vi "Make Up Setup Plot.vi"(4 "End Field":dbl format="%.2f", 5 "Start Field":dbl format="%.2f", 6 "Put in plot 1":bool, 7 "End X":i32, 8 "error in (no error)":errorcluster, 9 "Start X":i32, 10 "Plot 1 In":cluster{dbl[], dbl[]} {"?" format="%.2f"; "?" format="%.2f"}, 11 "Plot 2 In":cluster{dbl[], dbl[]} {"?" format="%.2f"; "?" format="%.2f"}) -> (0 "error out":errorcluster, 2 "Plot 1 Out":cluster{dbl[], dbl[]} {"?" format="%.2f"; "?" format="%.2f"}, 3 "Plot 2 Out":cluster{dbl[], dbl[]} {"?" format="%.2f"; "?" format="%.2f"})   [LabVIEW 2018, in "Multi Segment Waveform.xctl"]
doc: "Add a single ramp segment to one of two plots"
uses:
  Multi Segment Waveform.xctl
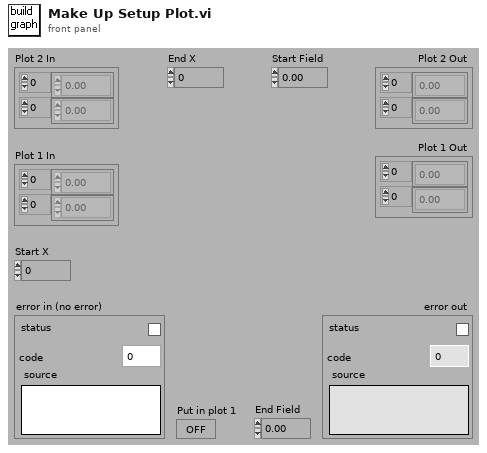
[diagram p1: front panel]
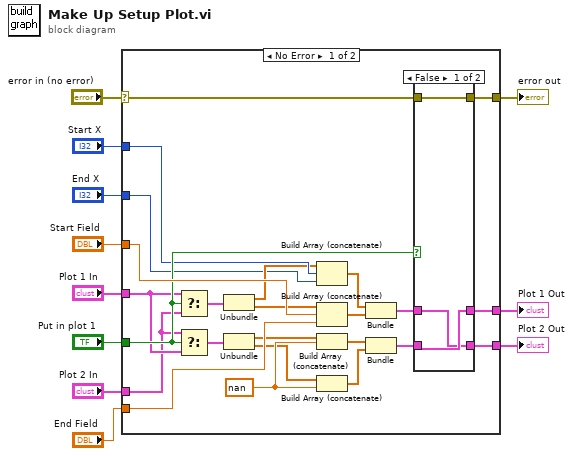
[diagram p0: block diagram]
diagram:
  n1 = case shown="No Error" "error in (no error)" {
    selector: "error in (no error)" -> [w13 w43]
    tunnel: [w35 w42] -> w11
    tunnel: [w34 _] -> w10
    tunnel: "End Field" -> [w33 _]
    tunnel: "Start Field" -> [w32 _]
    tunnel: "Put in plot 1" -> [w28 _]
    tunnel: "Plot 1 In" -> [w21 w42]
    tunnel: "Plot 2 In" -> [w20 _]
    tunnel: "Start X" -> [w17 _]
    tunnel: "End X" -> [w14 _]
    tunnel: [w12 w43] -> w1
    frame No Error {
      w25 = nan
      n2 = Select(t=w21, s=w28, f=w20) -> (s? t:f=w15:cluster{dbl[], dbl[]})
      n3 = Select(t=w20, s=w28, f=w21) -> (s? t:f=w22:cluster{dbl[], dbl[]})
      n4 = Unbundle(w15) -> (w16:dbl[], w31:dbl[])
      n5 = Unbundle(w22) -> (w23:dbl[], w24:dbl[])
      n6 = Build Array (concatenate)(w16, w17, w14) -> (w18:dbl[])
      n7 = Build Array (concatenate)(w31, w32, w33) -> (w19:dbl[])
      n8 = Build Array (concatenate)(w23, w25) -> (w26:dbl[])
      n9 = Build Array (concatenate)(w24, w25) -> (w27:dbl[])
      n10 = Bundle(w18, w19) -> (w30:cluster{dbl[], dbl[]})  [unwired: 1 out]
      n11 = Bundle(w26, w27) -> (w29:cluster{dbl[], dbl[]})  [unwired: 1 out]
      n12 = case shown="False" w28 {
        tunnel: w29 -> [w38 w41]
        tunnel: [w37 w41] -> w35
        tunnel: [w38 w40] -> w34
        tunnel: w30 -> [w37 w40]
        tunnel: w13 -> [w36 w39]
        tunnel: [w36 w39] -> w12
        frame False {
        }
        frame True {
        }
      }
    }
    frame Error {
    }
  }
  "Plot 2 Out" <- w11
  "Plot 1 Out" <- w10
  "error out" <- w1
